vi "RxBuffer.vi"(0 "RxData":u8[](array[numeric]), 3 "Clear?":bool, 5 "error in (no error)":errorcluster) -> (8 "RxData Raw":u8[](array[numeric]), 9 "DeviceParameters":T1 {"DevInfo"."ASICtrim" format="%02x"}, 10 "Dut Serial #":u32 format="%08d", 11 "LoadSensors":dbl[](array[numeric]), 12 "New Data Program":bool, 13 "Accelerometer":dbl[](array[numeric]), 14 "RxData Out":u16[](array[numeric]) format="%02x", 15 "DUT Serial Number":u32, 16 "CalData":dbl[][](array[numeric]), 17 "New Data":bool, 18 "Packet Check":bool, 19 "error out":errorcluster)   [LabVIEW 2015]
uses:
  Controls/DeviceInfo.ctl
  Controls/InfoPacket.ctl
  Controls/Gen2 FT Globals.vi
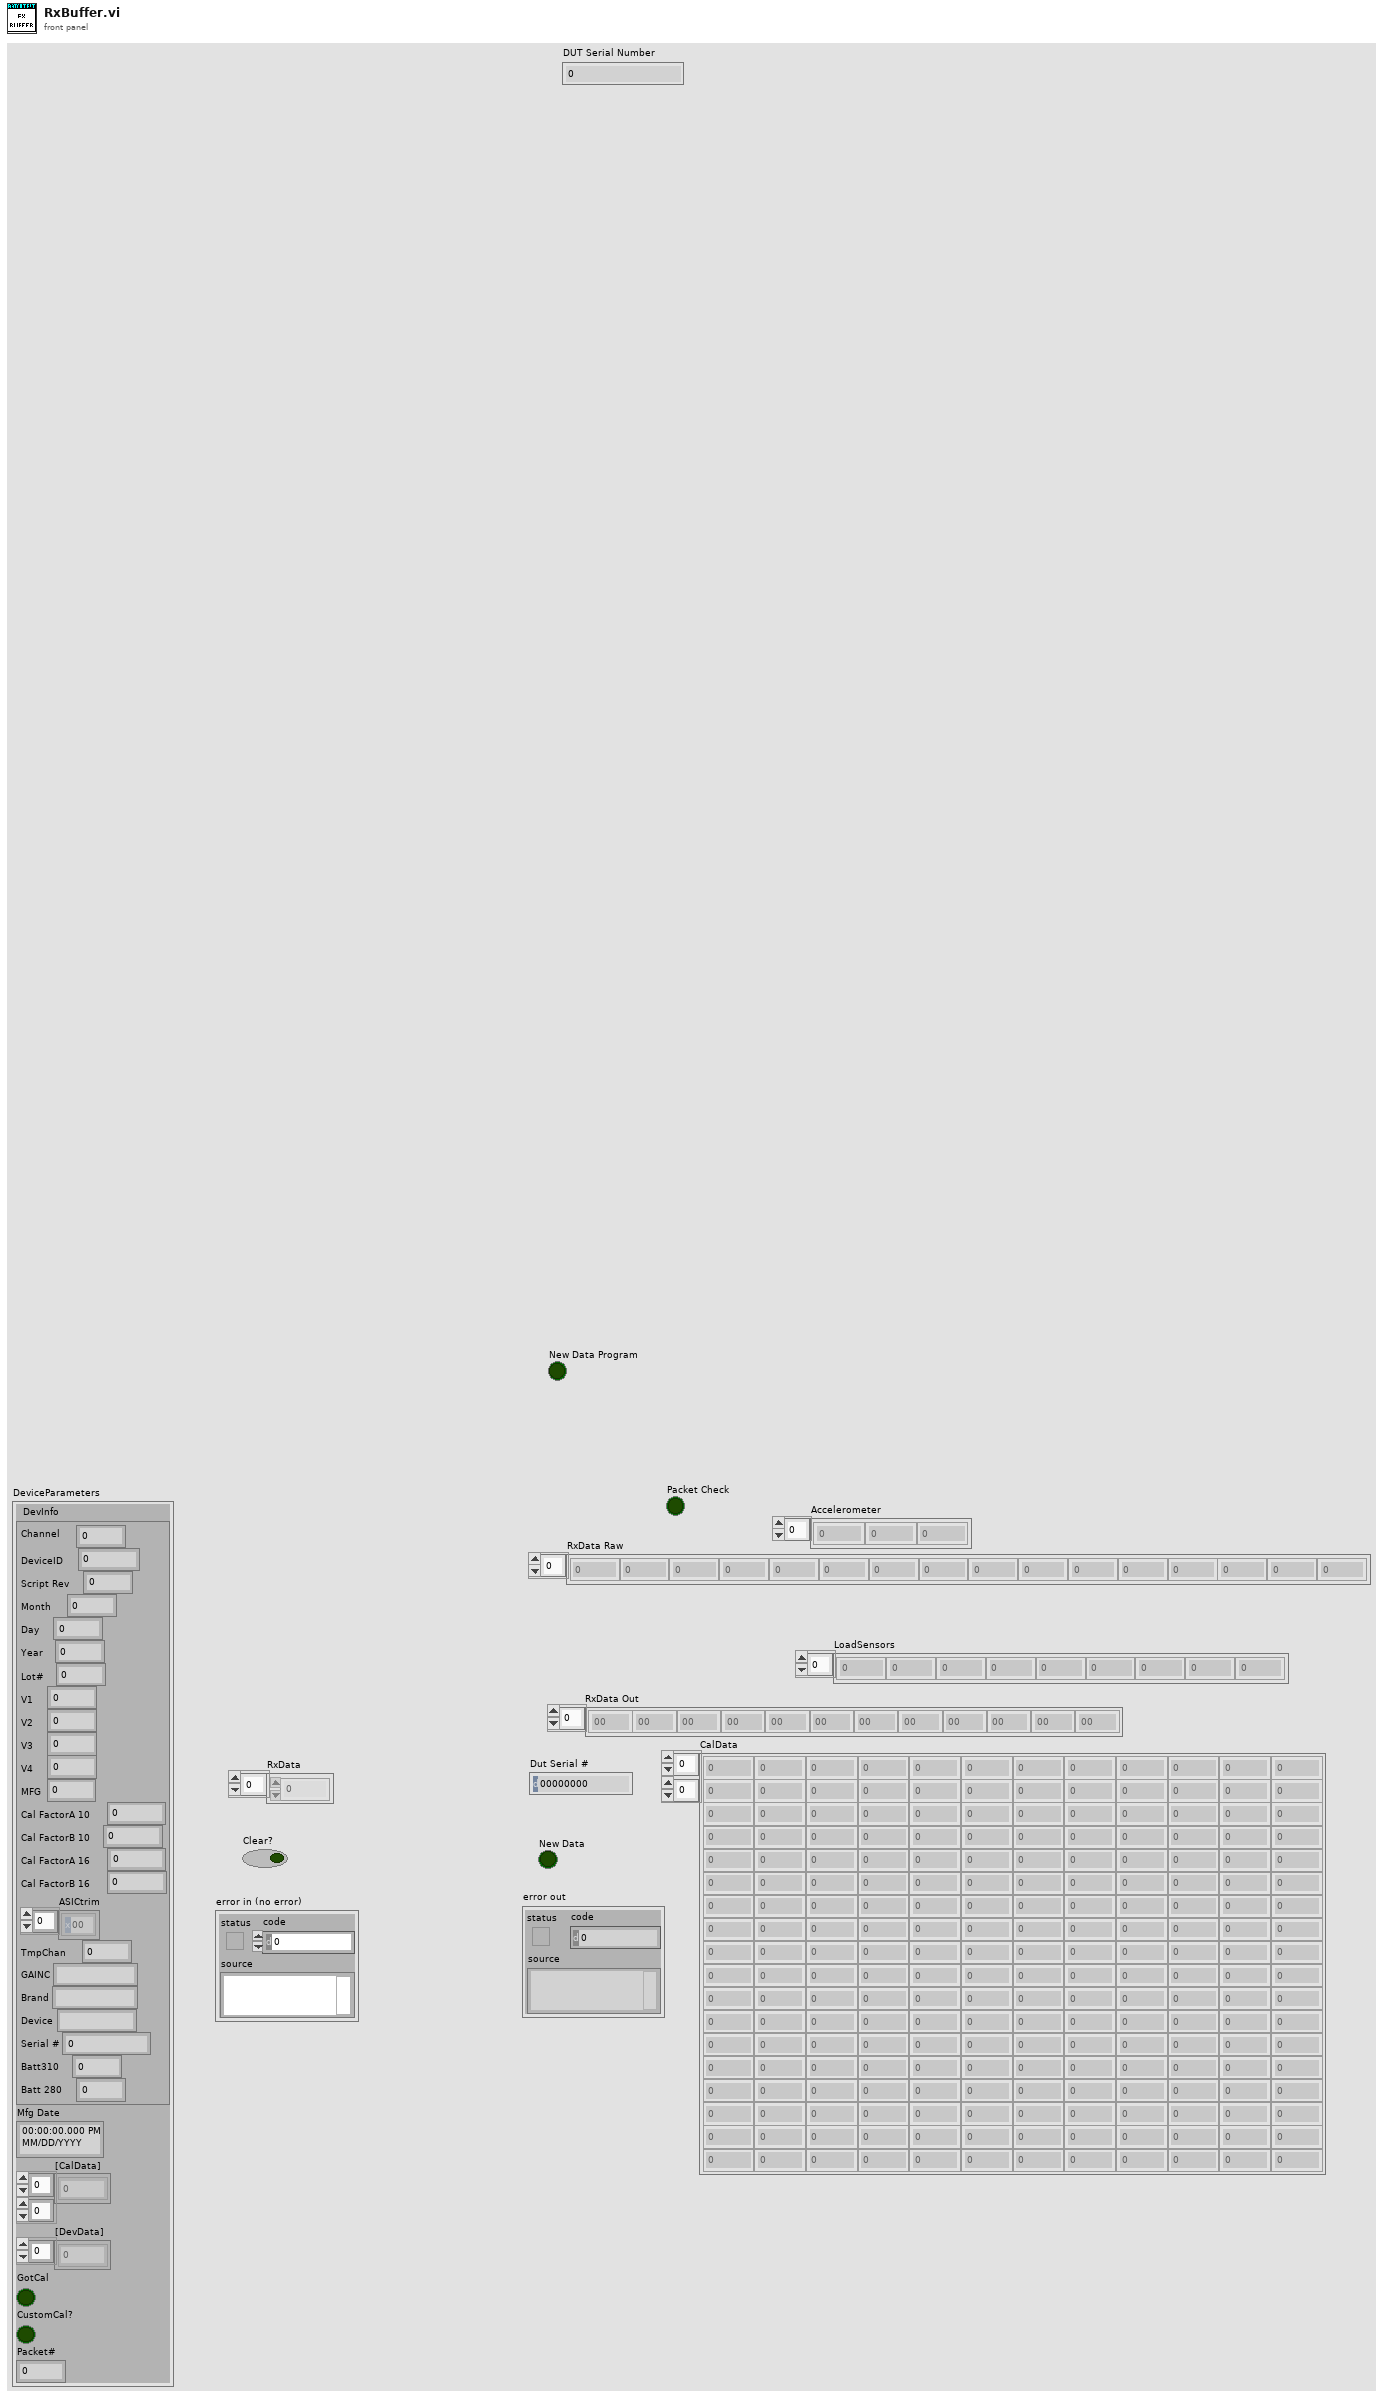
[diagram p1: front panel]
types:
  T1 = typedef "DeviceInfo.ctl" = cluster{"DevInfo":T2, "Mfg Date":timestamp, "[CalData]":u8[][], "[DevData]":u8[], "GotCal":bool, "CustomCal?":bool, "Packet#":i32}
  T2 = typedef "InfoPacket.ctl" = cluster{"Channel":u8, "DeviceID":u32, "Script Rev":u8, "Month":u8, "Day":u8, "Year":u8, "Lot#":u32, "V1":u16, "V2":u16, "V3":u16, "V4":u16, "MFG":u8, "Cal FactorA 10":u8, "Cal FactorB 10  ":u8, "Cal FactorA 16":u8, "Cal FactorB 16":u8, "ASICtrim":u8[], "TmpChan":u8, "GAINC":string, "Brand":string, "Device":string, "Serial #":u64, "Batt310":u16, "Batt 280":u16}
  T3 = typedef "LiveData.ctl" = cluster{"LoadSensors":dbl[], "Reference/Temperature 1":dbl, "Battery":dbl, "RefCalFactor":dbl, "StartingRef":dbl, "Raw USB Data":u16[], "ZeroedBattV":dbl, "AvgBufferFilled?":bool, "Accelerometer":dbl[], "Reference/Temperature 2":dbl}
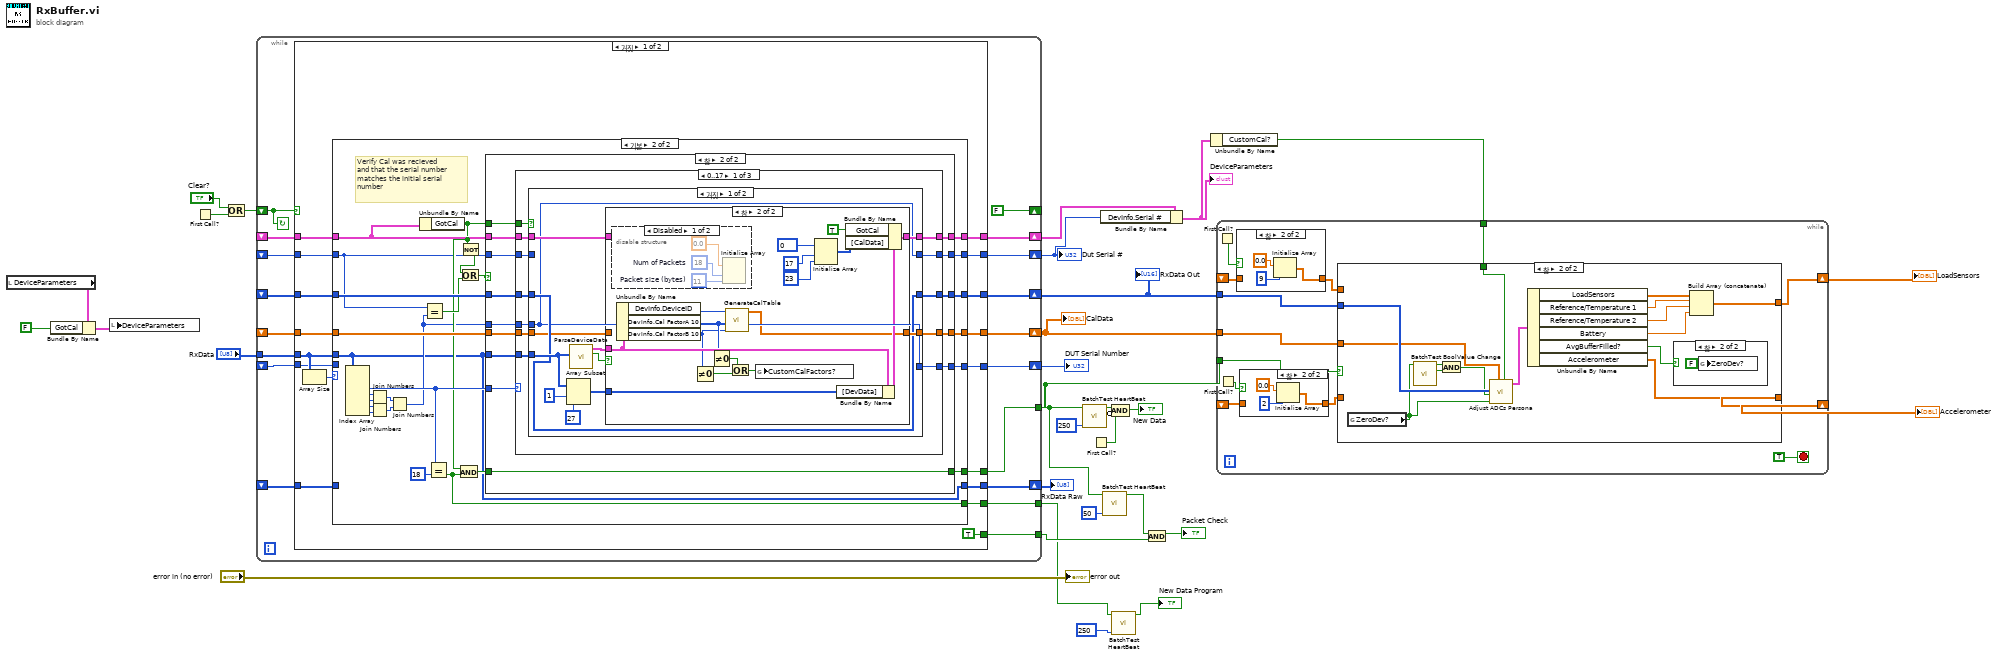
[diagram p0: block diagram]
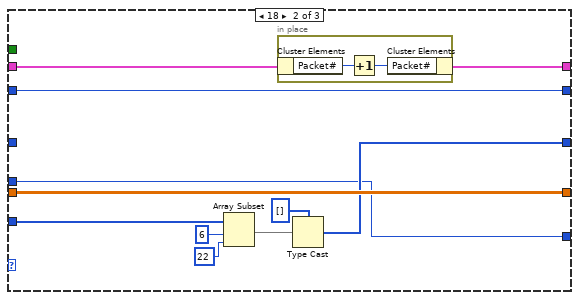
[diagram p11: hidden frame]
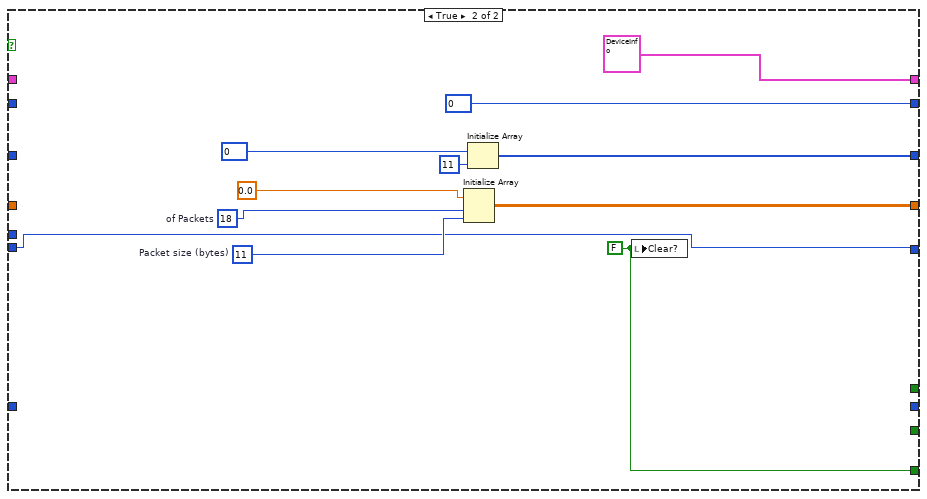
[diagram p13: hidden frame]
diagram:
  n1 = local read "DeviceParameters"() -> (w12:T1)
  n2 = Bundle By Name(cluster=w12, "GotCal"=FALSE) -> (w10:T1)
  n3 = local write "DeviceParameters"(w10) -> ()
  n4 = First Call?() -> (First Call?: T/F=w27:bool)
  n5 = Or(x="Clear?", y=w27) -> (x .or. y?=w28:bool)
  n6 = while {
    shift-right: [w47] -> w24
    shift-left: _ -> [w46]
    shift-right: [w45] -> w25
    shift-left: _ -> [w44]
    shift-right: [FALSE ("First Call?: T/F")] -> _
    shift-left: w28 -> [w48]
    tunnel: "RxData" -> [w42]
    shift-right: [w41] -> w14
    shift-left: _ -> [w40]
    shift-right: [w39] -> w16
    shift-left: _ -> [w38]
    shift-right: [w37] -> w22
    shift-left: _ -> [w36]
    tunnel: [w35] -> w8
    tunnel: [w34] -> w7
    shift-right: [w33] -> w4
    shift-left: _ -> [w32]
    tunnel: [w31] -> w2
    stop <- w48 continue-if-true
    n7 = case shown="거짓" w48 {
      tunnel: [w64 w195] -> w47
      tunnel: w46 -> [w65 _]
      tunnel: [w62 w194] -> w45
      tunnel: w44 -> [w63 _]
      tunnel: w42 -> [w61 _]
      tunnel: [w58 u32 0] -> w41
      tunnel: w40 -> [w59 _]
      tunnel: [w56 T1 {"DevInfo"={"Channel"=0, "DeviceID"=0, "Script Rev"=0, "Month"=0, "Day"=0, "Year"=0, "Lot#"=0, "V1"=0, "V2"=0, "V3"=0, "V4"=0, "MFG"=0, "Cal FactorA 10"=0, "Cal FactorB 10  "=0, "Cal FactorA 16"=0, "Cal FactorB 16"=0, "ASICtrim"=[], "TmpChan"=0, "GAINC"="", "Brand"="", "Device"="", "Serial #"=0, "Batt310"=0, "Batt 280"=0}, "Mfg Date"=timestamp(0 s since 1904-01-01), "[CalData]"=[], "[DevData]"=[], "GotCal"=FALSE, "CustomCal?"=FALSE, "Packet#"=0} ("Cluster")] -> w39
      tunnel: w38 -> [w57 _]
      tunnel: [w55 _] -> w37
      tunnel: w36 -> [w54 _]
      tunnel: [w53 _] -> w35
      tunnel: [TRUE ("Clear?") w186] -> w34
      tunnel: [w51 w185] -> w33
      tunnel: w32 -> [w50 w185]
      tunnel: [w49 _] -> w31
      frame False {
        n8 = Array Size(array=w61) -> (size(s)=w60:i32)
        n9 = case shown="기본" w60 {
          tunnel: w65 -> [w71 w97]
          tunnel: [w71 w96] -> w64
          tunnel: w63 -> [w70 w94]
          tunnel: [w70 w95] -> w62
          tunnel: w61 -> [_ w72]
          tunnel: w59 -> [w69 w76]
          tunnel: [w69 w93] -> w58
          tunnel: w57 -> [w68 w83]
          tunnel: [w68 w86] -> w56
          tunnel: [w67 w72] -> w55
          tunnel: w54 -> [w67 _]
          tunnel: [_ w77] -> w53
          tunnel: [w66 w74] -> w51
          tunnel: w50 -> [w66 _]
          tunnel: [_ w73] -> w49
          frame 0 {
          }
          frame Default {
            # "Verify Cal was recieved\nand that the serial number\nmatches the initial serial\nnumber"
            n10 = Index Array(array=w72) -> (element #2=w85:u8, element #3=w89:u8, element #4=w90:u8, element #5=w91:u8, element #6=w92:u8)  [unwired: 6 in, 1 out]
            n11 = Join Numbers(hi=w89, lo=w90) -> ((hi.lo)=w88:u16)
            n12 = Join Numbers(hi=w91, lo=w92) -> ((hi.lo)=w87:u16)
            n13 = Join Numbers(hi=w88, lo=w87) -> ((hi.lo)=w75:u32)
            n14 = Unbundle By Name(w83) -> ("GotCal"=w79:bool)
            n15 = Equal?(x=w76, y=w75) -> (x = y?=w80:bool)
            n16 = Equal?(x=w85, y=u8 18) -> (x = y?=w73:bool)
            n17 = And(x=w79, y=w73) -> (x .and. y?=w78:bool)
            n18 = Not(x=w79) -> (.not. x?=w81:bool)
            n19 = Or(x=w81, y=w80) -> (x .or. y?=w82:bool)
            n20 = case shown="참" w82 {
              tunnel: w97 -> [w101 w116]
              tunnel: [w101 w115] -> w96
              tunnel: [w100 w114] -> w95
              tunnel: w94 -> [w100 w113]
              tunnel: [w102 w112] -> w93
              tunnel: w72 -> [_ w111]
              tunnel: w76 -> [w102 w110]
              tunnel: w85 -> [_ w109]
              tunnel: w75 -> [w98 w108]
              tunnel: w83 -> [w99 w107]
              tunnel: [w99 w106] -> w86
              tunnel: w79 -> [_ w105]
              tunnel: w78 -> [_ w104]
              tunnel: [_ w104] -> w77
              tunnel: [w98 w103] -> w74
              frame False {
                # "Serial numbers do not match\nignore packet"
              }
              frame True {
                n21 = case shown="0..17" w109 {
                  tunnel: w116 -> [w119 _ w183]
                  tunnel: [w120 w171 w183] -> w115
                  tunnel: w111 -> [w127 w168 _]
                  tunnel: [w125 w177 w184] -> w114
                  tunnel: w113 -> [w121 w177 w184]
                  tunnel: w110 -> [w123 w176 w182]
                  tunnel: [w122 w176 w182] -> w112
                  tunnel: w108 -> [w128 w167 w180]
                  tunnel: w107 -> [w124 w170 w181]
                  tunnel: [w126 w169 w181] -> w106
                  tunnel: w105 -> [w118 _ _]
                  tunnel: [w117 w167 w180] -> w103
                  frame 0..17 {
                    n22 = case shown="거짓" w118 {
                      tunnel: w128 -> [w129 w162]
                      tunnel: w127 -> [w140 _]
                      tunnel: [w135 w166] -> w126
                      tunnel: [w134 w164] -> w125
                      tunnel: w124 -> [w132 w166]
                      tunnel: w123 -> [_ w165]
                      tunnel: [w129 w165] -> w122
                      tunnel: w121 -> [w131 w164]
                      tunnel: [w133 w163] -> w120
                      tunnel: w119 -> [w133 w163]
                      tunnel: [w129 w162] -> w117
                      frame False {
                        n23 = Array Subset(array=w140, index=1, length=27) -> (w136:u8[])
                        n24 = call "ParseDeviceData.vi"("Packet0"=w140) -> ("DataGood?"=w130:bool, "Cluster"=w139:T1)  [unwired: 8 in, 1 out]
                        n25 = case shown="참" w130 {
                          tunnel: w139 -> [_ w150]
                          tunnel: w136 -> [_ w157]
                          tunnel: [w142 w156] -> w135
                          tunnel: [w141 w148] -> w134
                          tunnel: w132 -> [w142 _]
                          tunnel: w131 -> [w141 _]
                          frame False {
                          }
                          frame True {
                            n26 = disable-structure shown="Disabled" {
                              frame Disabled {
                                w160 = 18  # Num of Packets
                                w161 = 11  # Packet size (bytes)
                                n27 = Initialize Array(0.0, w160, w161) -> ()  [unwired: 1 out]
                              }
                              frame Enabled {
                              }
                            }
                            n28 = Unbundle By Name(w150) -> ("DevInfo.DeviceID"=w149:u32, "DevInfo.Cal FactorA 10"=w147:u8, "DevInfo.Cal FactorB 10"=w146:u8)
                            n29 = Not Equal To 0?(x=w146) -> (x != 0?=w144:bool)
                            n30 = Not Equal To 0?(x=w147) -> (x != 0?=w145:bool)
                            n31 = call "GenerateCalTable.vi"("CalFactorB"=w146, "CalFactorA"=w147, "DeviceType"=w149) -> ("Array"=w148:dbl[][])  [unwired: 8 in]
                            n32 = Or(x=w145, y=w144) -> (x .or. y?=w143:bool)
                            n33 = global write "Gen2 FT Globals.vi" "CustomCalFactors?"(w143) -> ()
                            n34 = Initialize Array(u8 0, 17 ("dimension size"), 23 ("dimension size")) -> (w152:u8[][])
                            n35 = Bundle By Name(cluster=w150, "[DevData]"=w157) -> (w158:T1)
                            n36 = Bundle By Name(cluster=w158, "GotCal"=TRUE, "[CalData]"=w152) -> (w156:T1)
                          }
                        }
                      }
                      frame True {
                      }
                    }
                  }
                  frame 18 {
                    n37 = Array Subset(array=w168, index=6, length=22) -> (w175:u8[])
                    n38 = in-place {
                      n39 = in-place-cluster #1(w170) -> ("Packet#"=w179:i32)
                      n40 = Increment(x=w179) -> (x+1=w178:i32)
                      n41 = in-place-cluster #1("Packet#"=w178) -> (w169:T1)
                    }
                    n42 = Type Cast(type=u16[] [], x=w175) -> (*(type *) &x=w171:u16[])
                  }
                  frame Default {
                  }
                }
              }
            }
          }
        }
      }
      frame True {
        w186 = FALSE ("Clear?")
        w190 = 18  # of Packets
        w191 = 11  # Packet size (bytes)
        n43 = Initialize Array(0.0, w190, w191) -> (w194:dbl[][])
        n44 = Initialize Array(u16 0, 11 ("dimension size")) -> (w195:u16[])
        n45 = local write "Clear?"(w186) -> ()
      }
    }
  }
  "CalData" <- w25
  "Dut Serial #" <- w14
  "RxData Out" <- w24
  "RxData Raw" <- w22
  "DUT Serial Number" <- w4
  n46 = call "BatchTest HeartBeat.vi"("MaxTime"=u32 250, "Value In"=w8) -> ("Alive?"=w20:bool)  [unwired: 8 in, 1 out]
  n47 = First Call?() -> (First Call?: T/F=w18:bool)
  n48 = Bundle By Name(cluster=w16, "DevInfo.Serial #"=w14) -> (w15:T1)
  "DeviceParameters" <- w15
  n49 = call "BatchTest HeartBeat.vi"("MaxTime"=u32 50, "Value In"=w8) -> ("Alive?"=w6:bool)  [unwired: 8 in, 1 out]
  n50 = Compound Arithmetic op=AND(w20, invert w18) -> (→"New Data":bool)
  n51 = call "BatchTest HeartBeat.vi"("MaxTime"=u32 250, "Value In"=w2) -> ("Alive?"=→"New Data Program":bool)  [unwired: 8 in, 1 out]
  n52 = And(x=w6, y=w7) -> (x .and. y?=→"Packet Check":bool)
  n53 = Unbundle By Name(w15) -> ("CustomCal?"=w17:bool)
  n54 = while {
    tunnel: w8 -> [w208]
    tunnel: w25 -> [w207]
    tunnel: w24 -> [w206]
    shift-right: [w204] -> w23
    shift-left: _ -> [w201]
    tunnel: w17 -> [w200]
    shift-right: [w196] -> w13
    shift-left: _ -> [w197]
    stop <- TRUE stop-if-true
    n55 = First Call?() -> (First Call?: T/F=w203:bool)
    n56 = First Call?() -> (First Call?: T/F=w199:bool)
    n57 = case shown="참" w203 {
      tunnel: [w213 w215] -> w202
      tunnel: w201 -> [w213 _]
      frame False {
      }
      frame True {
        n58 = Initialize Array(0.0 ("element"), 9 ("dimension size")) -> (w215:dbl[])
      }
    }
    n59 = case shown="참" w199 {
      tunnel: [w209 w211] -> w198
      tunnel: w197 -> [w209 _]
      frame False {
      }
      frame True {
        n60 = Initialize Array(0.0 ("element"), 2 ("dimension size")) -> (w211:dbl[])
      }
    }
    n61 = case shown="참" w208 {
      tunnel: w206 -> [_ w225]
      tunnel: w207 -> [_ w224]
      tunnel: [w218 w231] -> w204
      tunnel: w202 -> [w218 _]
      tunnel: w200 -> [_ w220]
      tunnel: [w217 w226] -> w196
      tunnel: w198 -> [w217 _]
      frame False {
      }
      frame True {
        n62 = global read "Gen2 FT Globals.vi" "ZeroDev?"() -> (w221:bool)
        n63 = call "BatchTest BoolValue Change.vi"("Value In"=w221) -> ("Value Changed?"=w228:bool, "Value Out"=w227:bool)  [unwired: 7 in, 2 out]
        n64 = And(x=w227, y=w228) -> (x .and. y?=w222:bool)
        n65 = call "Adjust ADCs Persona.vi"("CustomCal?"=w220, "Original CalData"=w224, "Recal?"=w221, "Clear?"=w222, "Live Raw USB data"=w225) -> ("LiveData"=w219:T3)  [unwired: 6 in]
        n66 = Unbundle By Name(w219) -> ("LoadSensors"=w232:dbl[], "Reference/Temperature 1"=w230:dbl, "Reference/Temperature 2"=w229:dbl, "Battery"=w223:dbl, "AvgBufferFilled?"=w233:bool, "Accelerometer"=w226:dbl[])
        n67 = case shown="참" w233 {
          frame False {
          }
          frame True {
            n68 = global write "Gen2 FT Globals.vi" "ZeroDev?"(FALSE ("ZeroDev?")) -> ()
          }
        }
        n69 = Build Array (concatenate)(w232, w230, w229, w223) -> (w231:dbl[])
      }
    }
  }
  "LoadSensors" <- w23
  "Accelerometer" <- w13
  "error out" <- "error in (no error)"
